vi "DeployImage_Main.vi"(8 "error in (no error)":errorcluster, 11 "DevInfo":T1={"Hostname"="", "IPAddress"="", "MAC"="", "SerialNum"="", "Model"="", "Status"="", "FW"="", "OSDesc"="", "ImgTitle"="", "ImgDesc"="", "ImgVer"="", "ImgID"="", "IP Address Request Mode"=1, "SubnetMask"="", "Gateway"="", "DNSServer"=""} {"IP Address Request Mode" items=["Static"=1, "DHCP/Link-Local"=2, "Link-Local Only"=4, "DHCP Only"=8]}) -> (0 "error out":errorcluster)   [LabVIEW 2021]
uses:
  TypeDefs/DevInfo.ctl
  TypeDefs/DeployImageStates.ctl
  TypeDefs/AppImageProperties.ctl
  TypeDefs/FPGA_Properties_Element.ctl
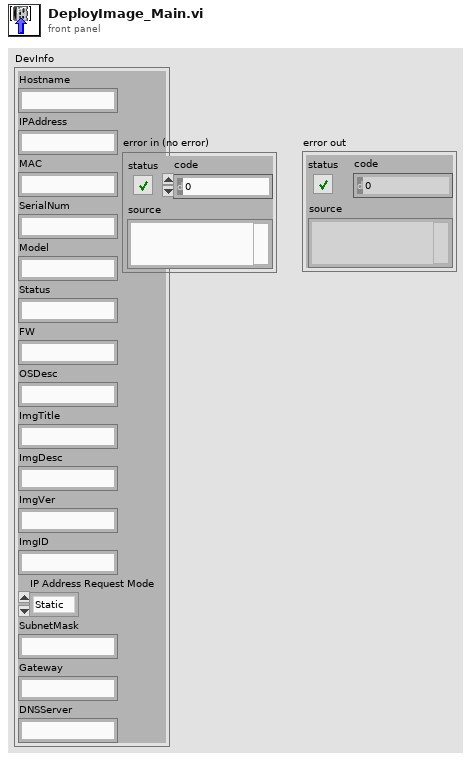
[diagram p1: front panel]
types:
  T1 = typedef "DevInfo.ctl" = cluster{"Hostname":string, "IPAddress":string, "MAC":string, "SerialNum":string, "Model":string, "Status":string, "FW":string, "OSDesc":string, "ImgTitle":string, "ImgDesc":string, "ImgVer":string, "ImgID":string, "IP Address Request Mode":i32, "SubnetMask":string, "Gateway":string, "DNSServer":string}
  T2 = typedef "AppImageProperties.ctl" = cluster{"Name":string, "Version":string, "Time":timestamp, "Description":string, "Key":string, "Chassis":string, "FPGA Properties":T3[], "Model":string, "Retrieve":string[], "Deploy":string[], "Installed Software":string[]}
  T3 = typedef "FPGA_Properties_Element.ctl" = cluster{"Resource Name":string, "Path":path}
  T4 = typedef "DeployImageStates.ctl" = enum16{"Select Image File", "Extract Image", "Display Image Info", "Deploy Image", "Clean Up", "Exit"}
  T5 = cluster{"Selected Image File":path, "AppImage Properties":T2}
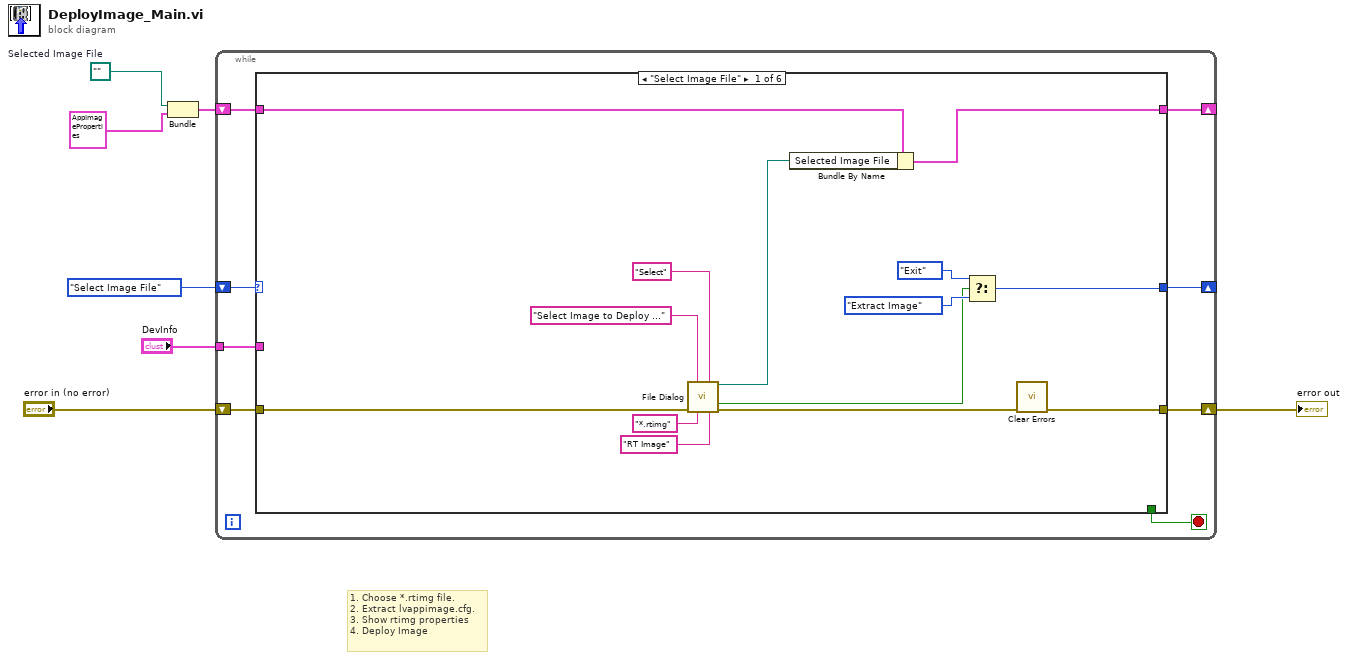
[diagram p0: block diagram]
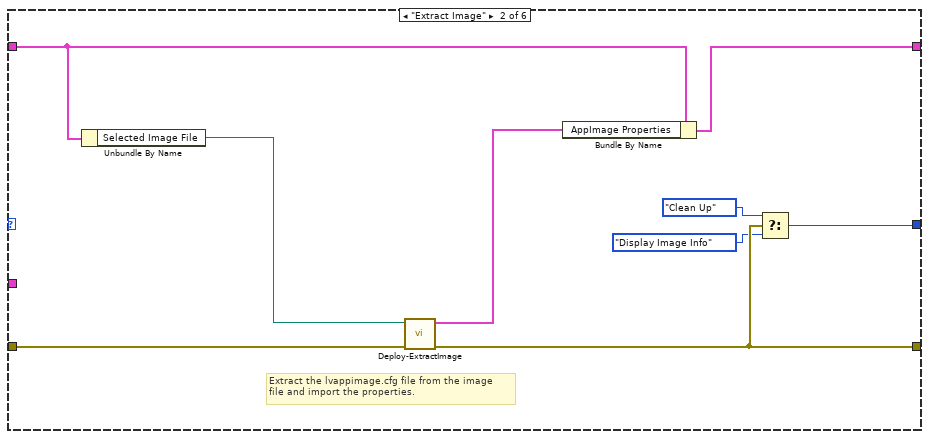
[diagram p2: hidden frame]
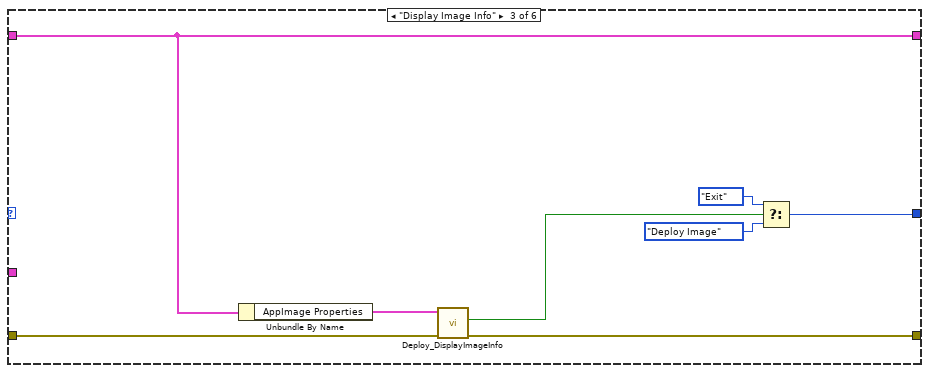
[diagram p3: hidden frame]
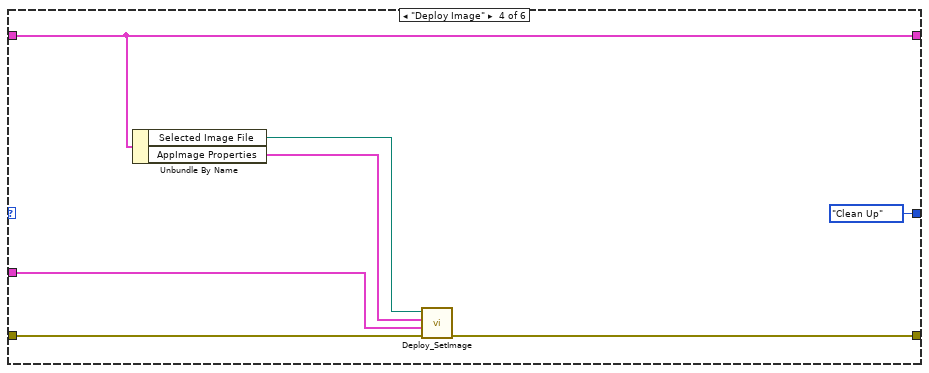
[diagram p4: hidden frame]
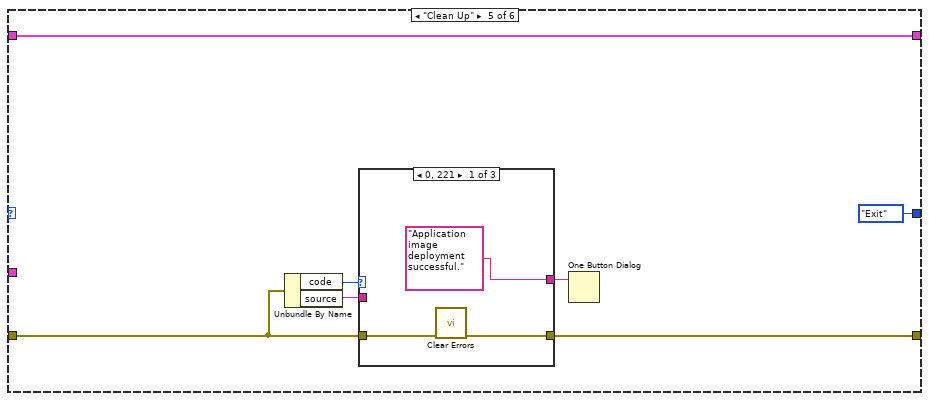
[diagram p5: hidden frame]
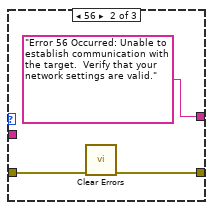
[diagram p6: hidden frame]
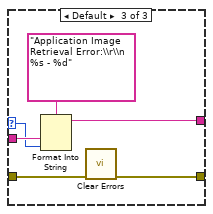
[diagram p7: hidden frame]
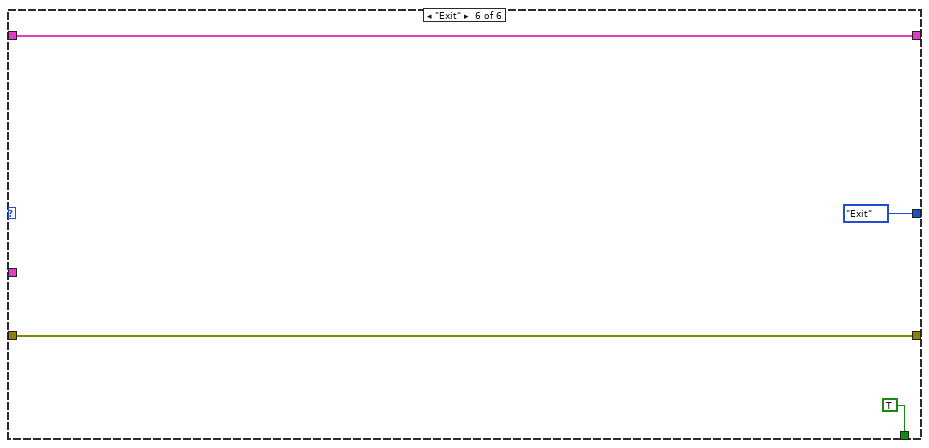
[diagram p8: hidden frame]
diagram:
  w4 = path ""  # Selected Image File
  # "1. Choose *.rtimg file.\n2. Extract lvappimage.cfg.\n3. Show rtimg properties\n4. Deploy Image"
  n1 = Bundle("Selected Image File"=w4, "AppImage Properties"=T2 {"Name"="", "Version"="", "Time"=timestamp(0 s since 1904-01-01), "Description"="", "Key"="", "Chassis"="", "FPGA Properties"=[], "Model"="", "Retrieve"=[], "Deploy"=[], "Installed Software"=[]}) -> (w3:T5)  [unwired: 1 in]
  n2 = while {
    shift-right: [w12] -> _
    shift-left: DeployImageStates."Select Image File" -> [w15]
    shift-right: [w13] -> w5
    shift-left: "error in (no error)" -> [w14]
    shift-right: [w10] -> _
    shift-left: w3 -> [w11]
    tunnel: "DevInfo" -> [w8]
    stop <- w9 stop-if-true
    n3 = case shown="\"Select Image File\"" w15 {
      tunnel: w14 -> [w26 w38 w46 w49 w57 w74]
      tunnel: [w20 w34 w45 w50 w56 w74] -> w13
      tunnel: [w22 w31 w41 DeployImageStates."Clean Up" DeployImageStates."Exit" DeployImageStates."Exit"] -> w12
      tunnel: w11 -> [w18 w35 w40 w52 w55 w75]
      tunnel: [w19 w36 w40 w52 w55 w75] -> w10
      tunnel: [_ _ _ _ _ TRUE] -> w9
      tunnel: w8 -> [_ _ _ w51 _ _]
      frame "Select Image File" {
        n4 = call "File Dialog"("prompt"="Select Image to Deploy ...", "button label"="Select" ("prompt"), "error in"=w26, "pattern (all files)"="*.rtimg", "pattern label"="RT Image") -> ("selected path"=w17:path, "cancelled"=w23:bool, "error out"=w21:errorcluster)  [unwired: 7 in, 1 out]
        n5 = Bundle By Name(cluster=w18, "Selected Image File"=w17) -> (w19:T5)
        n6 = Select(t=DeployImageStates."Exit", s=w23, f=DeployImageStates."Extract Image") -> (s? t:f=w22:T4)
        n7 = call <vilib>:"Clear Errors.vi"("error in (no error)"=w21) -> ("error out"=w20:errorcluster)  [unwired: 5 in, 1 out]
      }
      frame "Extract Image" {
        # "Extract the lvappimage.cfg file from the image\nfile and import the properties."
        n8 = Unbundle By Name(w35) -> ("Selected Image File"=w37:path)
        n9 = call "Deploy-ExtractImage.vi"("error in (no error)"=w38, "Selected Image File"=w37) -> ("error out"=w34:errorcluster, "AppImage Properties"=w30:T2)  [unwired: 8 in]
        n10 = Bundle By Name(cluster=w35, "AppImage Properties"=w30) -> (w36:T5)
        n11 = Select(t=DeployImageStates."Clean Up", s=w34, f=DeployImageStates."Display Image Info") -> (s? t:f=w31:T4)
      }
      frame "Display Image Info" {
        n12 = Unbundle By Name(w40) -> ("AppImage Properties"=w39:T2)
        n13 = call "Deploy_DisplayImageInfo.vi"("error in (no error)"=w46, "AppImage Properties"=w39) -> ("error out"=w45:errorcluster, "Cancelled?"=w42:bool)  [unwired: 8 in]
        n14 = Select(t=DeployImageStates."Exit", s=w42, f=DeployImageStates."Deploy Image") -> (s? t:f=w41:T4)
      }
      frame "Deploy Image" {
        n15 = Unbundle By Name(w52) -> ("Selected Image File"=w47:path, "AppImage Properties"=w48:T2)
        n16 = call "Deploy_SetImage.vi"("error in (no error)"=w49, "DevInfo"=w51, "AppImage Properties"=w48, "Selected Image File"=w47) -> ("error out"=w50:errorcluster)  [unwired: 7 in]
      }
      frame "Clean Up" {
        n17 = Unbundle By Name(w57) -> ("code"=w59:i32, "source"=w60:string)
        n18 = case shown="0, 221" w59 {
          selector: w59 -> [_ _ w69]
          tunnel: w60 -> [_ _ w72]
          tunnel: ["Application image deployment successful." ("source") "Error 56 Occurred: Unable to establish communication with the target.  Verify that your network settings are valid." ("source") w71] -> w58
          tunnel: [w61 w64 w67] -> w56
          tunnel: w57 -> [w62 w65 w68]
          frame 0, 221 {
            n19 = call <vilib>:"Clear Errors.vi"("error in (no error)"=w62) -> ("error out"=w61:errorcluster)  [unwired: 5 in, 1 out]
          }
          frame 56 {
            n20 = call <vilib>:"Clear Errors.vi"("error in (no error)"=w65) -> ("error out"=w64:errorcluster)  [unwired: 5 in, 1 out]
          }
          frame Default {
            n21 = Format Into String(format string="Application Image Retrieval Error:\\r\\n %s - %d", w72, w69) -> (resulting string=w71:string)  [unwired: 2 in, 1 out]
            n22 = call <vilib>:"Clear Errors.vi"("error in (no error)"=w68) -> ("error out"=w67:errorcluster)  [unwired: 5 in, 1 out]
          }
        }
        n23 = One Button Dialog(message=w58) -> ()  [unwired: 2 out]
      }
      frame "Exit" {
      }
    }
  }
  "error out" <- w5
